vi "Created Remove.vi"(9 "Created Alias":string, 10 "Addresses DVR in":refnum<data-value>) -> (0 "error out":errorcluster, 2 "Addresses DVR out":refnum<data-value>)   [LabVIEW 2021, in "jettl.lvlib" / "Addresses.lvlib" / "Addresses.lvclass"]
uses:
  Addresses.lvclass
  Addresses.lvclass/Addresses.ctl
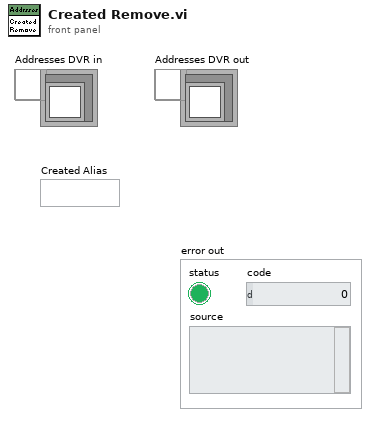
[diagram p1: front panel]
types:
  T1 = typedef "jettl.lvlib/Addresses.lvlib/Created.ctl" = map{string, refnum<class "Msg Type Strategy.lvclass">}
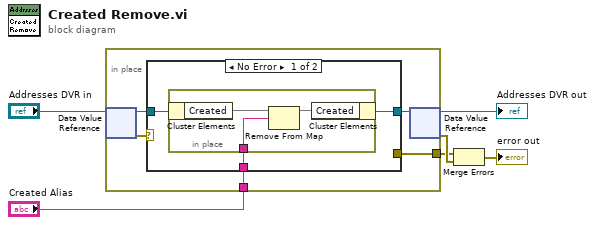
[diagram p0: block diagram]
diagram:
  n1 = in-place {
    in-place-border: [w11] -> w2
    in-place-border: "Created Alias" -> [w8]
    n2 = in-place-dvr #1("Addresses DVR in") -> (w9:refnum<class "Addresses.lvclass">, w10:errorcluster)
    n3 = case shown="No Error" w10 {
      selector: w10 -> [_ w19]
      tunnel: w9 -> [w13 w18]
      tunnel: [_ w19] -> w11
      tunnel: w8 -> [w14 _]
      tunnel: [w12 w18] -> w7
      frame No Error {
        n4 = in-place {
          in-place-border: w14 -> [w17]
          n5 = in-place-cluster #2(w13) -> ("Created"=w16:T1)
          n6 = Remove From Map(10:w17, 11:w16) -> (3:w15:T1)  [unwired: 2 out]
          n7 = in-place-cluster #2("Created"=w15) -> (w12:refnum<class "Addresses.lvclass">)
        }
      }
      frame Error {
      }
    }
    n8 = in-place-dvr #1(w7) -> (→"Addresses DVR out":refnum<data-value>, w3:errorcluster)
  }
  n9 = Merge Errors(w2, w3) -> (→"error out":errorcluster)
